vi "add_cp.vi"(8 "FFT size":u32=256, 9 "CP length":u32=64, 11 "time_samples":cdb[](array[numeric])) -> (3 "cp ofdm symbol":cdb[](array[numeric]))   [LabVIEW 2014]
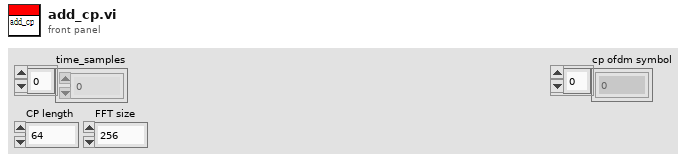
[diagram p1: front panel]
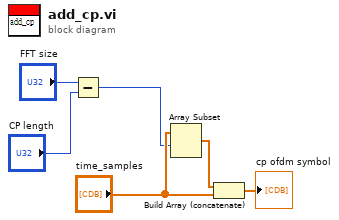
[diagram p0: block diagram]
diagram:
  n1 = Subtract(x="FFT size", y="CP length") -> (x-y=w1:u32)
  n2 = Array Subset(array="time_samples", index=w1) -> (w4:cdb[])  [unwired: 1 in]
  n3 = Build Array (concatenate)(w4, "time_samples") -> (→"cp ofdm symbol":cdb[])
